vi "ex5.vi"() -> ()   [LabVIEW 2022 SP3]
panel:
  out "U8 result":u8
  out "U32":u32
  in  "I8":i8
  in  "U32":u32
  out "U8 result":u8
  in  "I32":i32
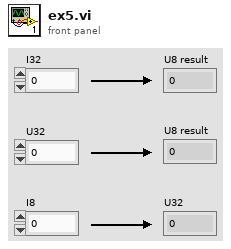
[diagram p1: front panel]
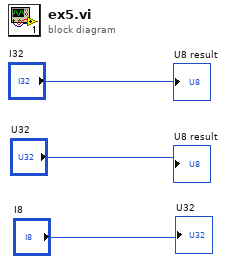
[diagram p0: block diagram]
diagram:
  "U8 result" <- "I32"
  "U32" <- "I8"
  "U8 result" <- "U32"
